vi "port_read.vi"(8 "error in (no error)":errorcluster, 11 "VISA Refnum in":refnum<visa-resource-name>) -> (0 "error out":errorcluster, 2 "reply":string, 3 "VISA Refnum out":refnum<visa-resource-name>)   [LabVIEW 2024]
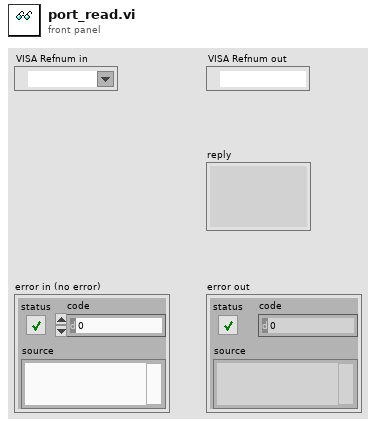
[diagram p1: front panel]
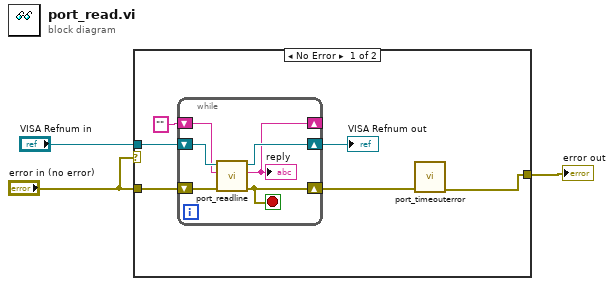
[diagram p0: block diagram]
diagram:
  n1 = case shown="No Error" "error in (no error)" {
    tunnel: "error in (no error)" -> [w7 w16]
    tunnel: "VISA Refnum in" -> [w6 _]
    tunnel: [w5 w16] -> w2
    frame No Error {
      n2 = while {
        shift-right: [w13] -> w8
        shift-left: w6 -> [w15]
        shift-right: [w11] -> w4
        shift-left: w7 -> [w14]
        shift-right: [w10] -> _
        shift-left: "" -> [w12]
        stop <- w11 stop-if-true
        n3 = call "port_readline.vi"("error in (no error)"=w14, "String in"=w12, "VISA Refnum in"=w15) -> ("error out"=w11:errorcluster, "reply"=w10:string, "VISA Refnum out"=w13:refnum<visa-resource-name>)  [unwired: 6 in]
        "reply" <- w10
      }
      "VISA Refnum out" <- w8
      n4 = call "port_timeouterror.vi"("error in (no error)"=w4) -> ("error out"=w5:errorcluster)  [unwired: 10 in]
    }
    frame Error {
    }
  }
  "error out" <- w2
